vi "Test MQTT-2.2.2-2.vi"(8 "error in (no error)":errorcluster) -> (0 "error out":errorcluster)   [LabVIEW 2013]
uses:
  <vilib>/addons/_JKI Toolkits/Caraya/classes/Test/Test.lvclass
  <vilib>/LabVIEW Open Source Project/MQTT Control Packets/Control Packets/CONNECT/CONNECT.lvclass
  <vilib>/LabVIEW Open Source Project/MQTT Control Packets/Control Packets/ControlPacket/ControlPacket.lvclass
  <vilib>/addons/_JKI Toolkits/Caraya/classes/Assert/Assert.lvclass
  <vilib>/LabVIEW Open Source Project/MQTT Connection/MQTT_Connection/Connection/Connection.lvclass
panel:
  out "connected":bool
  out "error out 2":errorcluster
  out "timed out":bool
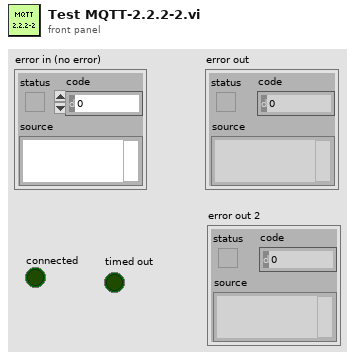
[diagram p1: front panel]
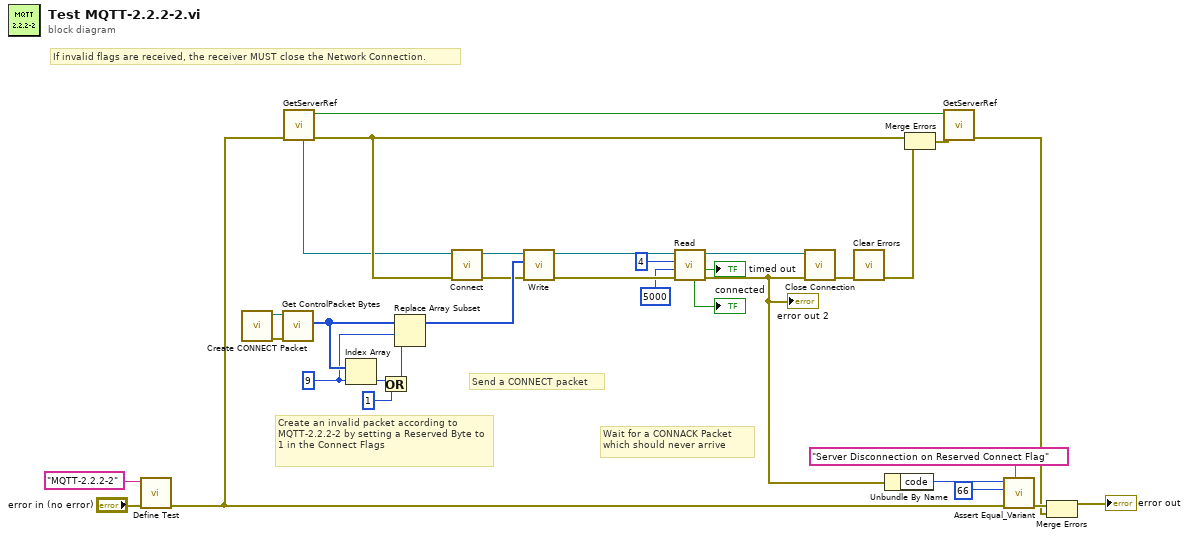
[diagram p0: block diagram]
diagram:
  w23 = 9 ("index")
  # "Wait for a CONNACK Packet\nwhich should never arrive"
  # "Create an invalid packet according to MQTT-2.2.2-2 by setting a Reserved Byte to 1 in the Connect Flags"
  # "Send a CONNECT packet"
  # "If invalid flags are received, the receiver MUST close the Network Connection."
  n1 = call <vilib>:"Define Test.vi"("error in (no error)"="error in (no error)", "Label (VI Title)"="MQTT-2.2.2-2") -> ("error out"=w4:errorcluster)  [unwired: 9 in]
  n2 = call <vilib>:"Create CONNECT Packet.vi"() -> ("error out"=w30:errorcluster, "CONNECT"=w31:refnum<class "CONNECT.lvclass">)  [unwired: 9 in, 1 out]
  n3 = call <vilib>:"Get ControlPacket Bytes.vi"("error in (no error)"=w30, "ControlPacket"=w31) -> ("Bytes Stream"=w25:u8[])  [unwired: 6 in, 3 out]
  n4 = call "GetServerRef.vi"("error in"=w4) -> ("error out"=w7:errorcluster, "Created"=w8:bool, "Connection Config"=w2:refnum<class "Connection.lvclass">)  [unwired: 7 in, 1 out]
  n5 = Index Array(array=w25, index=w23) -> (element=w27:u8)
  n6 = Or(x=w27, y=u8 1) -> (x .or. y?=w22:u8)
  n7 = Replace Array Subset(array=w25, new element=w22, index=w23) -> (w24:u8[])
  n8 = call <vilib>:"Connect.vi"("error in (no error)"=w7, "Connection in"=w2) -> ("error out"=w9:errorcluster, "Connection out"=w10:refnum<class "Connection.lvclass">)  [unwired: 8 in]
  n9 = call <vilib>:"Write.vi"("error in (no error)"=w9, "Bytes"=w24, "Connection in"=w10) -> ("error out"=w28:errorcluster, "Connection"=w29:refnum<class "Connection.lvclass">)  [unwired: 7 in]
  n10 = call <vilib>:"Read.vi"("error in (no error)"=w28, "timeout (2000 ms)"=5000 ("timeout ms (25000)"), "bytes to read (100)"=4 ("bytes to read"), "TCPConnection in"=w29) -> ("error out"=w13:errorcluster, "timed out"=→"timed out":bool, "TCPConnection out"=w21:refnum<class "Connection.lvclass">, "connected"=→"connected":bool)  [unwired: 3 in, 1 out]
  "error out 2" <- w13
  n11 = call <vilib>:"Close Connection.vi"("error in (no error)"=w13, "Connection in"=w21) -> ("error out"=w16:errorcluster)  [unwired: 8 in, 1 out]
  n12 = call <vilib>:"Clear Errors.vi"("error in (no error)"=w16) -> ("error out"=w12:errorcluster)  [unwired: 6 in]
  n13 = Unbundle By Name(w13) -> ("code"=w18:i32)
  n14 = Merge Errors(w7, w12) -> (w5:errorcluster)
  n15 = call "GetServerRef.vi"("error in"=w5, "Destroy (F)"=w8) -> ("error out"=w6:errorcluster)  [unwired: 6 in, 3 out]
  n16 = call <vilib>:"Assert Equal_Variant.vi"("Label"="Server Disconnection on Reserved Connect Flag", "error in (no error)"=w4, "Y"=66 ("code"), "X"=w18) -> ("error out"=w20:errorcluster)  [unwired: 7 in]
  n17 = Merge Errors(w20, w6) -> (→"error out":errorcluster)
